vi "animate.vi"() -> ()   [LabVIEW 2009]
uses:
  <vilib>/imath/engines/lvmath2/RunTimeEngine/ErrorHandling/NIMS_Finalize Error.vi
  <vilib>/imath/engines/lvmath2/RunTimeEngine/Parser/MC_Version.vi
  <vilib>/imath/engines/lvmath2/RunTimeEngine/NodeEndStatement/NIMS_NodeEndStatement_Output.vi
  <instcachedir>/0/NIMS_NodeEndStatement_Output_53EC0D466D134D7ABD903AC30B43404B.lvgen/NIMS_NodeEndStatement_Output_53EC0D466D134D7ABD903AC30B43404B_002.vi
  <vilib>/imath/engines/lvmath2/RunTimeEngine/BuiltInFunctions/linramp/NIMS_linramp.vi
  <vilib>/imathl/engines/lvmath/Functions/Error Handling/Create Error.vi
  <vilib>/imath/engines/lvmath2/RunTimeEngine/BuiltInFunctions/zeros/NIMS_M=zeros(I32,I32).vi
  <vilib>/imath/engines/lvmath2/RunTimeEngine/BuiltInFunctions/length/NIMS_length(GV).vi
  <instcachedir>/0/NIMS_length(GV)_08A3D13377FD4E4B96F5795FBF3698FA.lvgen/NIMS_length(GV)_08A3D13377FD4E4B96F5795FBF3698FA_000.vi
  <vilib>/imath/engines/lvmath2/RunTimeEngine/RangeToken/NIMS_Range_R3 - Float.vi
  <instcachedir>/0/NIMS_Range_R3 - Float_A37A80F5CD394C078DF94272B0675D0B.lvgen/NIMS_Range_R3 - Float_A37A80F5CD394C078DF94272B0675D0B_000.vi
  <vilib>/imath/engines/lvmath2/RunTimeEngine/ReplaceToken/NIMS_Replace - Assignment Check M(_,$)=VorM.vi
  <instcachedir>/0/NIMS_Replace - Assignment Check M(_,$)=VorM_3CB70357EF10473EBB509A04A4D02BC4.lvgen/NIMS_Replace - Assignment Check M(_,$)=VorM_3CB70357EF10473EBB509A04A4D02BC4_001.vi
  <vilib>/imath/engines/lvmath2/RunTimeEngine/ReplaceToken/NIMS_Replace - Size Check M(_,$)=VorM.vi
  <instcachedir>/0/NIMS_Replace - Size Check M(_,$)=VorM_EDDD90DB9294407A90551280BA264F99.lvgen/NIMS_Replace - Size Check M(_,$)=VorM_EDDD90DB9294407A90551280BA264F99_001.vi
  <vilib>/imath/engines/lvmath2/RunTimeEngine/ReplaceToken/NIMS_Replace - Check Row.vi
  <instcachedir>/0/NIMS_Replace - Check Row_C1FA588AB93341698A6951F0E3D02595.lvgen/NIMS_Replace - Check Row_C1FA588AB93341698A6951F0E3D02595_001.vi
  <vilib>/imath/engines/lvmath2/RunTimeEngine/CommandStatement/MC_CommandStatement_break.vi
panel:
  out "Animation":dbl[](graph)
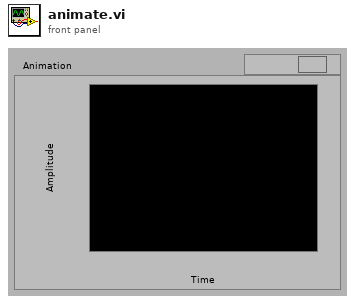
[diagram p1: front panel]
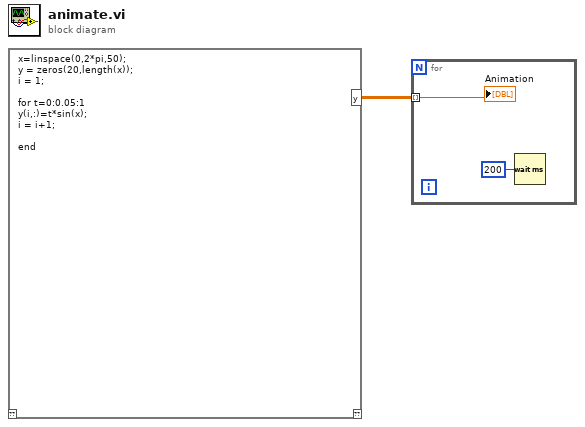
[diagram p0: block diagram]
diagram:
  n1 = mathscript code="x=linspace(0,2*pi,50);\ny = zeros(20,length(x));\ni = 1;\n\nfor t=0:0.05:1\ny(i,:)=t*sin(x);\ni = i+1;\n\nend"() -> ("y"=w1:dbl[][])  [unwired: 1 in, 1 out]
  n2 = for {
    tunnel: w1 -> [w3] mode=indexing
    n3 = Wait (ms)(milliseconds to wait=u32 200) -> ()  [unwired: 1 out]
    "Animation" <- w3
  }
